vi "getMode.vi"(8 "error in (no error)":errorcluster, 11 "ethernetSupply in":refnum<class "ethernetSupply.lvclass">) -> (0 "error out":errorcluster, 2 "mode":enum16{"current", "voltage"}[](array[ring]), 3 "ethernetSupply out":refnum<class "ethernetSupply.lvclass">)   [LabVIEW 2011, in "Tools.lvlib" / "DatabaseHelpers.lvlib" / "ethernetSupply.lvclass"]
uses:
  ethernetSupply.lvclass
  ethernetSupply.lvclass/ethernetSupply.ctl
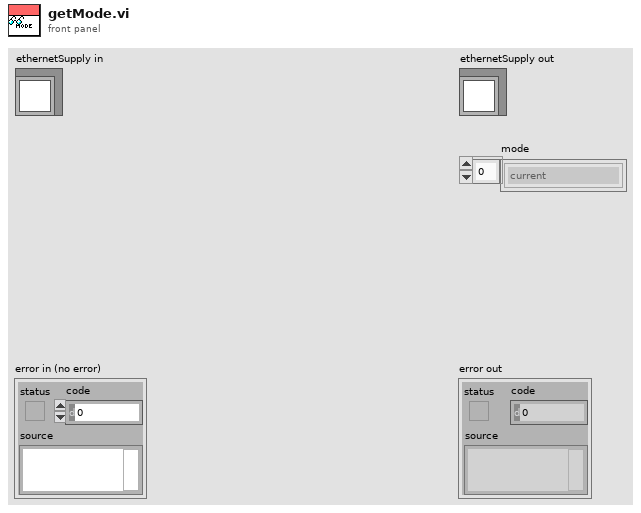
[diagram p1: front panel]
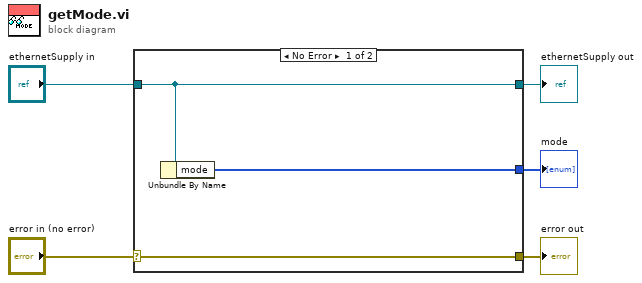
[diagram p0: block diagram]
diagram:
  n1 = case shown="No Error" "error in (no error)" {
    selector: "error in (no error)" -> [w8 w9]
    tunnel: [w8 w9] -> w4
    tunnel: [w7 w10] -> w2
    tunnel: "ethernetSupply in" -> [w7 w10]
    tunnel: [w6 _] -> w1
    frame No Error {
      n2 = Unbundle By Name(w7) -> ("mode"=w6:enum16{"current", "voltage"}[])
    }
    frame Error {
    }
  }
  "error out" <- w4
  "ethernetSupply out" <- w2
  "mode" <- w1
